vi "Dev_LCR_E4980_Real_time_2022-04-05-RM_v15.vi"() -> ()   [LabVIEW 2021]
doc: "This example shows how to configure a measurement and take readings."
uses:
  <vilib>/Platform/TimedLoop/XDataNode/timing_clust.ctl
  <vilib>/Platform/TimedLoop/XDataNode/nitl_modes.ctl
  <vilib>/Platform/TimedLoop/XDataNode/wakeup.ctl
  <vilib>/Utility/file.llb/Write Delimited Spreadsheet (DBL).vi
  <vilib>/platform/TimedLoop/XDataNode/XDataNode.xnode
  <instrlib>/Agilent E4980/Agilent E4980.lvlib
  <vilib>/Platform/TimedLoop/XDataNode/XDNodeRunTimeDep.lvlib
panel:
  out "?":dbl format="%<%H:%M:%S>t"
  in  "Addition Volume (uL)":string="Unspecified"
  in  "Tab Control":T1(tab)
  in  "Alarm Preaddittion (Sec)":dbl=30.0
  in  "User":string="Richard Murray"
  out "Param 4":string
  out "Param 3":string
  in  "Addittion Time (mins)":dbl=5.0
  in  "Sound Notifications":bool=TRUE
  in  "Analyte":string="Unspecified"
  in  "?":bool
  out "Param 2":string
  out "Param 1":string
  out "Loop":i32
  out "Array":dbl[][](array[numeric])
  in  "Polling rate (ms)":dbl=100.0
  out "Time (s)":dbl format="%<%H:%M:%S>t"
  in  "Duration (mins)":dbl=120.0
  in  "Averaging Factor (1)":i32=1
  in  "Measurement Time (1: Med)":u16(ring)=2 items=["Short", "Medium", "Long"]
  in  "Signal Level (1.0 V)":dbl=1.0
  in  "Signal Type (0: Voltage)":u16(ring) items=["Voltage", "Current"]
  in  "Signal Frequency (1000 Hz)":dbl=1000.0
  in  "Enable Auto Range (T:Enable)":bool=TRUE
  in  "Manual Impedance Range (3: 100 Ohms)":i32(ring)=3 items=["100m", "1", "10", "100", "300", "1K", "3K", "10K", "30K", "100K"]
  in  "Function (3: Cp-Rp)":u16(ring)=6 items=["Cp-D", "Cp-Q", "Cp-G", "Cp-Rp", "Cs-D", "Cs-Q", "Cs-Rs", "Lp-D", "Lp-Q", "Lp-G", "Lp-Rp", "Lp-Rdc", "Ls-D", "Ls-Q", "Ls-Rs", "Ls-Rdc", "R-X", "Z-thd", "Z-thr", "G-B", "Y-thd", "Y-thr", "Vdc-Idc"]
  out "Primary Parameter":dbl
  out "Secondary Parameter":dbl
  in  "VISA resource name (LCR)":refnum<visa-resource-name>="LCR"
  out "Primary Param Chart":dbl(graph)
  out "Secondary Param Chart":dbl(graph)
  # "(c) 2007-2015 National Instruments.  ALL RIGHTS RESERVED\nModified for specific use by Richard Murray 2022."
  # "Equipment Definitions"
  # "Monitoring Panel"
  # "Real Time"
  # "Post Data View"
  # "Time (s)"
  # "Param 1"
  # "Param 2"
  # "Measurement Mode"
  # "Meta Data"
  # "Define equipment source, needs keysight connection expert to know the GPIB address, but this can be changed to any given ALIAS address e.g. LCR, which is the default here.\n\nLeave \"Auto Range\" on, this allows the equipment to determine the value of allowed impedence, Manual impedacne can be set if this is disabled.\n\nSound notifications are on by default, chimming at the end of the run, and at a predetermined time (30s, before an addittion is due)"
  # "Select the pair of parameters to record (default is Cp-Rp)\nSelect the controlled parameter Voltage/Current, which is driving the process\nSelect the applied magnitude of the control parameter (e.g. 1V)\nChoose the measuring frequency (e.g. 1kHz)\nSelect the averaging factor, number of measurements made per point\nChoose the measurement time, longer is more accurate, but less time fidelity (equipment defined factor)\nChoose, in minutes how long you would like to record for\nChoose the polling rate, the rate at which the equipment is queired for a new data point, depends on the measurement time & averaging factor"
  # "User: Meta date populated to output file\nAnalyte: Meta date populated to output file\nAddittion Time: Meta date populated to output file, and sets an alarm timer, to remind you to insert analyte\nAlarm Preaddition: How long before the addittion you want the alarm"
  # "Real Time: Shows the data as it is recorded, including the loop number, time in seconds and the targetted parameters\n\nPost Data view: Shows the full recorded data after the process has been stopped"
  # "STOP and SAVE has been implemented to allow you to escape the run time of the process while preserving the data in the output file."
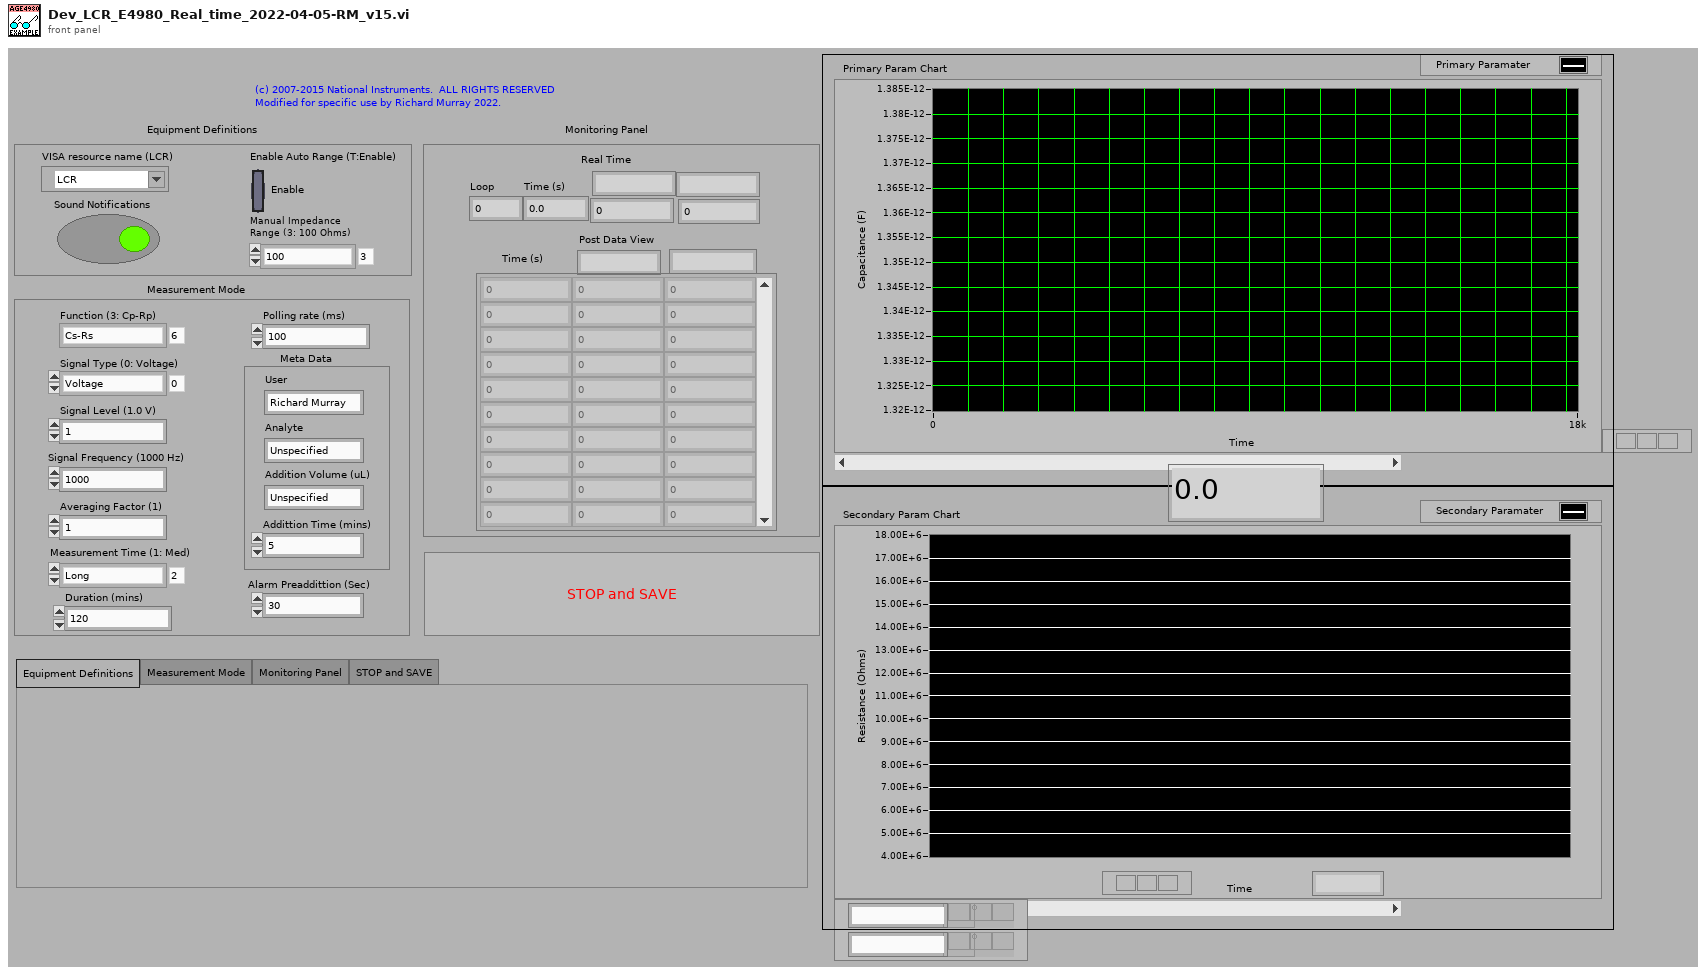
[diagram p1: front panel]
types:
  T1 = enum32{"Equipment Definitions", "Measurement Mode", "Monitoring Panel", "STOP and SAVE"}
  T2 = enum16{"open", "replace", "create", "open or create", "replace or create", "replace or create with confirmation"}
  T3 = typedef "XDNodeRunTimeDep.lvlib/timing_clust.ctl" = cluster{"Expected End [f-1]":u64, "Actual End [f-1]":u64, "Finished Late? [f-1]":bool, "Expected End [i-1]":u64, "Actual End [i-1]":u64, "Finished Late? [i-1]":bool, "Expected Start [i]":u64, "Actual Start [i]":u64, "Expected Start [f]":u64, "Actual Start [f]":u64, "Source Name":string, "Structure Name":string, "Period":i64, "Deadline":i64, "Offset":i64, "Start":i64, "Priority":i32, "Timeout":i32, "Mode":T4, "Wakeup Reason":T5, "Error":errorcluster, "Source Type":string, "Secondary Source Type":string, "Global End Time":u64, "Global Start Time":u64, "Frame Duration":u64, "Iteration Duration":u64, "Assigned CPU":i32, "I/O Scan Engine Mode":u32}
  T4 = typedef "XDNodeRunTimeDep.lvlib/nitl_modes.ctl" = enum32{"No Change", "Process missed periods, maintain original phase", "Discard missed periods, maintain original phase", "Process missed periods, ignore original phase", "Discard missed periods, ignore original phase"}
  T5 = typedef "XDNodeRunTimeDep.lvlib/wakeup.ctl" = enum32{"Normal", "Aborted", "Asynchronous wakeup", "Timing source error", "Timed loop error", "Timeout"}
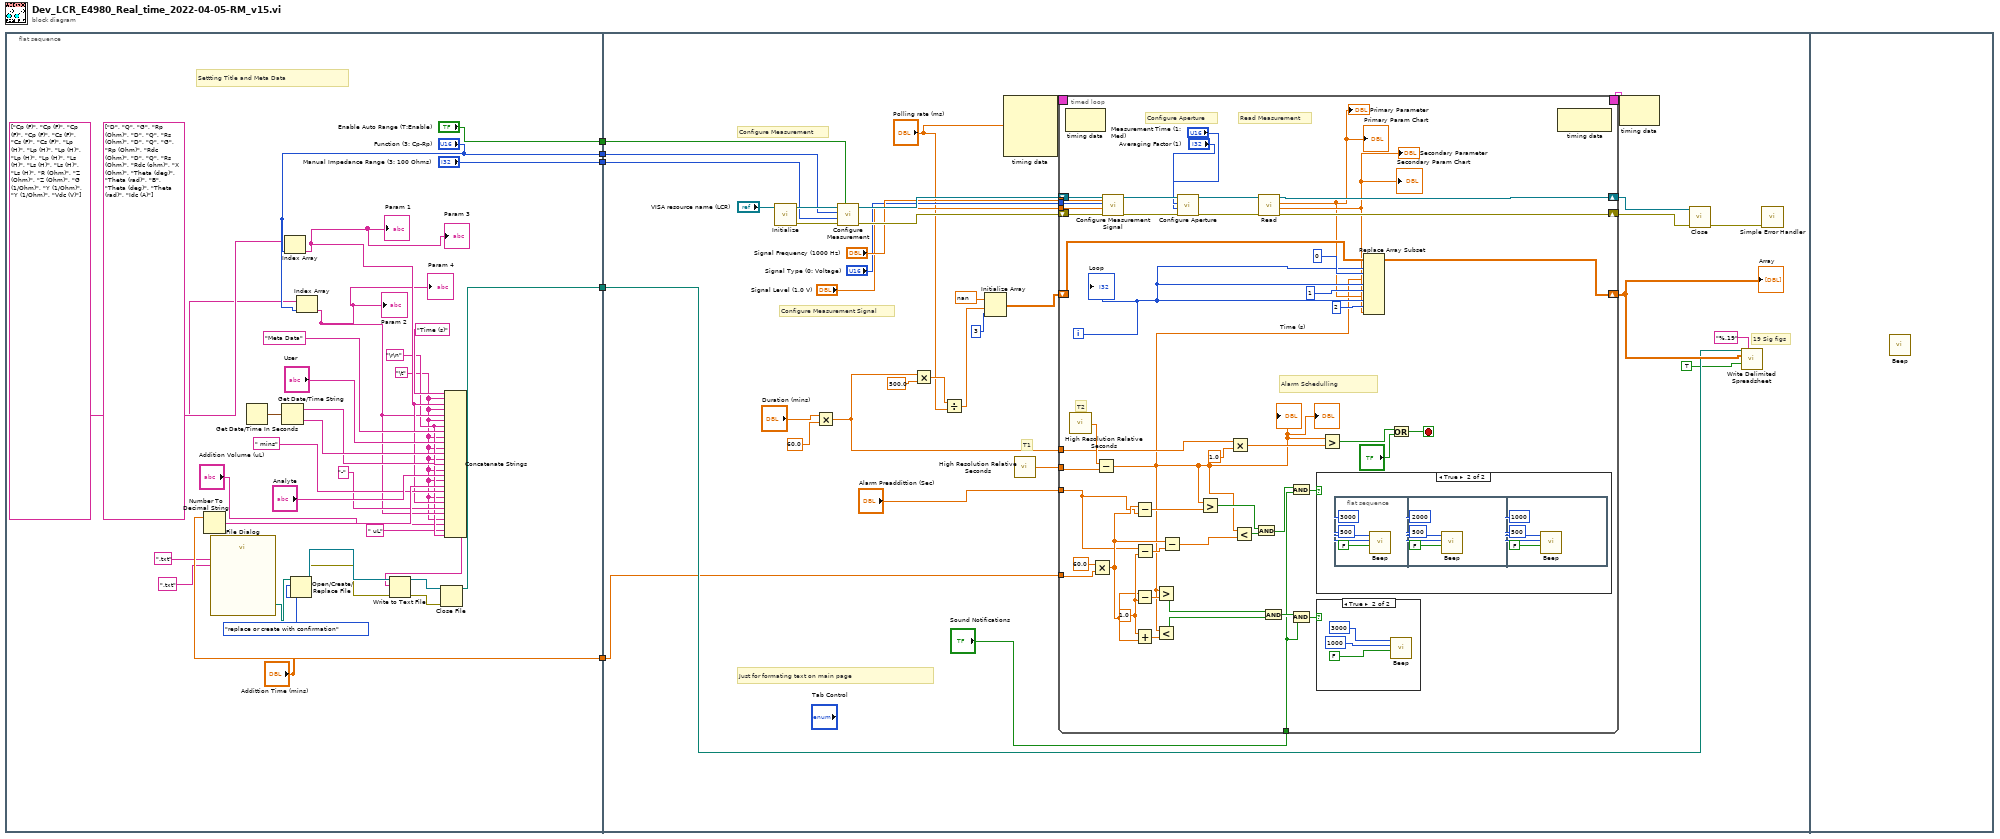
[diagram p0: block diagram]
diagram:
  n1 = flat-sequence {
    tunnel: [w27] -> w5
    tunnel: ["Enable Auto Range (T:Enable)"] -> w4
    tunnel: ["Function (3: Cp-Rp)"] -> w3
    tunnel: ["Manual Impedance Range (3: 100 Ohms)"] -> w2
    tunnel: ["Addittion Time (mins)"] -> w1
    tunnel: w5 -> [w49]
    tunnel: w4 -> [w48]
    tunnel: w3 -> [w47]
    tunnel: w2 -> [w46]
    tunnel: w1 -> [w39]
    frame #0 {
      w8 = "\t"
      w9 = "\r\n"
      # "Settting Title and Meta Data"
      n2 = Number To Decimal String(number="Addittion Time (mins)") -> (decimal integer string=w17:string)  [unwired: 1 in]
      n3 = call "File Dialog"("pattern (all files)"=".txt", "pattern label"=".txt") -> ("selected path"=w11:path)  [unwired: 10 in, 3 out]
      n4 = Get Date/Time In Seconds() -> (seconds since 1Jan1904=w24:timestamp)
      n5 = Get Date/Time String(seconds (now)=w24) -> (date string=w19:string, time string=w20:string)  [unwired: 2 in]
      n6 = Index Array(array=string[] ["Cp (F)", "Cp (F)", "Cp (F)", "Cp (F)", "Cs (F)", "Cs (F)", "Cs (F)", "Lp (H)", "Lp (H)", "Lp (H)", "Lp (H)", "Lp (H)", "Ls (H)", "Ls (H)", "Ls (H)", "Ls (H)", "R (Ohm)", "Z (Ohm)", "Z (Ohm)", "G (1/Ohm)", "Y (1/Ohm)", "Y (1/Ohm)", "Vdc (V)"], index="Function (3: Cp-Rp)") -> (element=w15:string)
      "Param 1" <- w15
      "Param 3" <- w15
      n7 = Open/Create/Replace File(file path (use dialog)=w11, operation (0:open)=T2."replace or create with confirmation") -> (refnum out=w33:refnum<file>, error out=w32:errorcluster)  [unwired: 4 in, 1 out]
      n8 = Index Array(array=string[] ["D", "Q", "G", "Rp (Ohm)", "D", "Q", "Rs (Ohm)", "D", "Q", "G", "Rp (Ohm)", "Rdc (Ohm)", "D", "Q", "Rs (Ohm)", "Rdc (ohm)", "X (Ohm)", "Theta (deg)", "Theta (rad)", "B", "Theta (deg)", "Theta (rad)", "Idc (A)"], index="Function (3: Cp-Rp)") -> (element=w13:string)
      "Param 2" <- w13
      "Param 4" <- w13
      n9 = Concatenate Strings("Time (s)" ("string"), w8, w15, w8, w13, w8, w9, "Meta Data" ("string"), w8, "User", w8, w20, w8, w19, w8, "Analyte", w8, w17, " mins" ("string"), w8, w15, "-" ("string"), w13, w8, "Addition Volume (uL)", " uL" ("string"), w9) -> (w28:string)
      n10 = Write to Text File(file (use dialog)=w33, text=w28, error in=w32) -> (refnum out=w30:refnum<file>, error out=w31:errorcluster)  [unwired: 1 in, 1 out]
      n11 = Close File(refnum=w30, error in=w31) -> (path=w27:path)  [unwired: 1 out]
    }
    frame #1 {
      # "Just for formating text on main page"
      # "19 Sig figs"
      # "T1"
      # "Configure Measurement Signal"
      # "Configure Measurement"
      n12 = call <instrlib>:"Initialize.vi"("VISA resource name"="VISA resource name (LCR)") -> ("error out"=w67:errorcluster, "VISA resource name out"=w68:refnum<visa-resource-name>)  [unwired: 9 in]
      n13 = Multiply(x="Duration (mins)", y=60.0) -> (x*y=w42:dbl)
      n14 = call <instrlib>:"Configure Measurement.vi"("Enable Auto Range (T:Enable)"=w48, "error in (no error)"=w67, "Manual Impedance Range (3: 100 Ohms)"=w46, "Function (0: Cp-D)"=w47, "VISA resource name"=w68) -> ("error out"=w62:errorcluster, "VISA resource name out"=w63:refnum<visa-resource-name>)  [unwired: 5 in]
      n15 = Multiply(x=w42, y=500.0) -> (x*y=w54:dbl)
      n16 = Divide(x=w54, y="Polling rate (ms)") -> (x/y=w40:dbl)
      n17 = Initialize Array(nan, w40, 3 ("dimension size")) -> (w56:dbl[][])
      n18 = node-c288("Polling rate (ms)") -> (w71:T3)  [unwired: 3 in]
      n19 = call <vilib>:"High Resolution Relative Seconds.vi"() -> ("relative seconds"=w58:dbl)
      n20 = timed-loop {
        timing: w71 -> [_]
        timing-out: [_] -> w70
        tunnel: "Signal Frequency (1000 Hz)" -> [w112]
        tunnel: "Signal Type (0: Voltage)" -> [w111]
        tunnel: "Signal Level (1.0 V)" -> [w110]
        shift-right: [w120] -> w66
        shift-left: w63 -> [w118]
        shift-right: [w119] -> w65
        shift-left: w62 -> [w117]
        tunnel: w58 -> [w104]
        shift-right: [w102] -> w51
        shift-left: w56 -> [w103]
        tunnel: w42 -> [w101]
        tunnel: "Sound Notifications" -> [w77]
        tunnel: w39 -> [w76]
        tunnel: "Alarm Preaddittion (Sec)" -> [w73]
        i -> [w99]
        stop <- w93 stop-if-true
        w75 = 1.0 ("x")
        # "Alarm Schedulling"
        # "T2"
        # "Configure Aperture"
        # "Read Measurement"
        n21 = node-c288() -> ()  [unwired: 1 in, 1 out]
        n22 = call <vilib>:"High Resolution Relative Seconds.vi"() -> ("relative seconds"=w105:dbl)
        n23 = Multiply(x=60.0, y=w76) -> (x*y=w74:dbl)
        n24 = Subtract(x=w105, y=w104) -> (x-y=w72:dbl)
        "Time (s)" <- w72
        "?" <- w72
        n25 = call <instrlib>:"Configure Measurement Signal.vi"("Signal Frequency (1000 Hz)"=w112, "error in (no error)"=w117, "Signal Level (1.0 V)"=w110, "Signal Type (0: Voltage)"=w111, "VISA resource name"=w118) -> ("error out"=w115:errorcluster, "VISA resource name out"=w116:refnum<visa-resource-name>)  [unwired: 5 in]
        n26 = Subtract(x=w74, y=w73) -> (x-y=w90:dbl)
        n27 = Subtract(x=w74, y=w75) -> (x-y=w81:dbl)
        n28 = Add(x=w75, y=w74) -> (x+y=w79:dbl)
        n29 = Subtract(x=w73, y=w75) -> (x-y=w84:dbl)
        n30 = Greater?(x=w72, y=w81) -> (0:w80:bool)
        n31 = Less?(x=w72, y=w79) -> (x < y?=w78:bool)
        n32 = Subtract(x=w74, y=w84) -> (x-y=w87:dbl)
        n33 = call <instrlib>:"Configure Aperture.vi"("error in (no error)"=w115, "Averaging Factor (1)"="Averaging Factor (1)", "Measurement Time (1: Medium)"="Measurement Time (1: Med)", "VISA resource name"=w116) -> ("error out"=w113:errorcluster, "VISA resource name out"=w114:refnum<visa-resource-name>)  [unwired: 6 in]
        n34 = Greater?(x=w72, y=w90) -> (0:w89:bool)
        n35 = Multiply(x=w101, y=1.0) -> (x*y=w106:dbl)
        n36 = Less?(x=w72, y=w87) -> (x < y?=w88:bool)
        n37 = And(x=w89, y=w88) -> (x .and. y?=w86:bool)
        n38 = call <instrlib>:"Read.vi"("error in (no error)"=w113, "VISA resource name"=w114) -> ("error out"=w119:errorcluster, "Secondary Parameter"=w96:dbl, "Primary Parameter"=w95:dbl, "VISA resource name out"=w120:refnum<visa-resource-name>)  [unwired: 6 in]
        "Primary Parameter" <- w95
        "Secondary Parameter" <- w96
        "Secondary Param Chart" <- w96
        "Primary Param Chart" <- w95
        n39 = And(x=w80, y=w78) -> (x .and. y?=w83:bool)
        n40 = And(x=w86, y=w77) -> (x .and. y?=w85:bool)
        n41 = And(x=w83, y=w77) -> (x .and. y?=w82:bool)
        n42 = case shown="True" w85 {
          frame False {
          }
          frame True {
            n43 = flat-sequence {
              frame #0 {
                n44 = call <vilib>:"Beep.vi"("use system alert? (T)"=FALSE, "duration (msec)"=u32 500, "frequency (Hz)"=u32 3000) -> ()  [unwired: 9 in]
              }
              frame #1 {
                n45 = call <vilib>:"Beep.vi"("use system alert? (T)"=FALSE, "duration (msec)"=u32 500, "frequency (Hz)"=u32 2000) -> ()  [unwired: 9 in]
              }
              frame #2 {
                n46 = call <vilib>:"Beep.vi"("use system alert? (T)"=FALSE, "duration (msec)"=u32 500, "frequency (Hz)"=u32 1000) -> ()  [unwired: 9 in]
              }
            }
          }
        }
        n47 = case shown="True" w82 {
          frame False {
          }
          frame True {
            n48 = call <vilib>:"Beep.vi"("use system alert? (T)"=FALSE, "duration (msec)"=u32 1000, "frequency (Hz)"=u32 3000) -> ()  [unwired: 9 in]
          }
        }
        n49 = Greater?(x=w72, y=w106) -> (0:w94:bool)
        n50 = Replace Array Subset(array=w103, new element #1=w72, index (row) #1=w99, index (col) #1=0 ("disabled index (row)"), new element #2=w95, index (row) #2=w99, index (col) #2=1 ("disabled index (col)"), new element #3=w96, index (row) #3=w99, index (col) #3=2 ("disabled index (col)")) -> (w102:dbl[][])
        n51 = Or(x=w94, y="?") -> (x .or. y?=w93:bool)
        n52 = node-c288() -> ()  [unwired: 1 in, 1 out]
        "Loop" <- w99
      }
      "Array" <- w51
      n53 = node-c288(w70) -> ()  [unwired: 1 out]
      n54 = call <instrlib>:"Close.vi"("error in (no error)"=w65, "VISA resource name"=w66) -> ("error out"=w64:errorcluster)  [unwired: 9 in]
      n55 = call-poly <vilib>:"Write Delimited Spreadsheet.vi"("file path (dialog if empty)"=w49, "format (%.3f)"="%.19", "2D data"=w51, "append to file? (new file:F)"=TRUE) -> ()  [unwired: 10 in, 2 out]
      n56 = call <vilib>:"Simple Error Handler.vi"("error in (no error)"=w64) -> ()  [unwired: 4 in, 5 out]
    }
    frame #2 {
      n57 = call <vilib>:"Beep.vi"() -> ()  [unwired: 12 in]
    }
  }
